vi "Bitfile EST Interfaces.vi"(11 "Version":T1) -> (2 "IP Types":T2[](array[typedef]), 3 "IP Interface":variant[](array[variant]))   [LabVIEW 2019, in "Engine Simulation Toolkit System Explorer.lvlib"]
uses:
  Engine Simulation Toolkit System Explorer.lvlib
  Shared/IP Interface Enum.ctl
  Shared/Bitfile EST Version.ctl
  Shared/Engine Simulation Toolkit Shared.lvlib
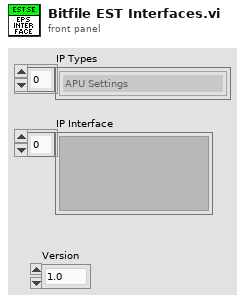
[diagram p1: front panel]
types:
  T1 = typedef "Engine Simulation Toolkit Shared.lvlib/Bitfile EST Version.ctl" = enum16{"1.0", "1.1", "1.2", "1.3", "1.4"}
  T2 = typedef "Engine Simulation Toolkit Shared.lvlib/IP Interface Enum.ctl" = enum16{"APU Settings", "APU Shared Settings", "APU Output", "APU Input", "Analog Replay Settings", "Analog Replay Load Input", "Analog Replay Input", "ETiming Capture Output", "ETiming Meas Settings", "ETiming Meas Output", "Digital PatGen Settings", "Digital PatGen Input", "Digital PatGen Load Input", "Knock Sensor Input", "Knock Sensor Settings", "Knock Cyl Input", "Knock Cyl Settings", "Dir Speed Input", "Dir Speed Settings", "Dir Speed Load Input", "APU Go"}
  T3 = cluster{"acceleration":fxp<+,18,-20>, "max cycle":fxp<+,2,2>, "enable accel":bool}
  T4 = cluster{"acceleration":fxp<+,18,-20>, "enable accel":bool}
  T5 = cluster{"cycle start":fxp<+,2,2>, "crank start":u16, "stuck limit":fxp<+,18,18>}
  T6 = cluster{"start":fxp<+,17,17>, "stuck limit":fxp<+,18,18>}
  T7 = cluster{"crank":u16, "cycle":u16, "actual speed":fxp<+/-,23,2>}
  T8 = cluster{"desired speed":fxp<+/-,23,2>, "reset":bool}
  T9 = cluster{"ReverseNegate":bool, "CycleAngle":bool, "SpeedThreshold":fxp<+/-,23,2>, "AOBelowThreshold":i16}
  T10 = cluster{"Data":i16[], "LoadOffset":u16, "Done":bool}
  T11 = cluster{"Offset":i16, "VScaleSlope":fxp<+,18,6>, "VScaleIntercept":fxp<+/-,18,3>}
  T12 = cluster{"Start":u16, "End":u16, "Duration (tics)":fxp<+,18,18>, "Event present":bool}
  T13 = cluster{"max":u16, "min":u16, "active high":bool, "wrap":bool, "full window":bool}
  T14 = cluster{"max":u16, "min":u16, "active high":bool, "wrap":bool}
  T15 = cluster{"stuck active":bool, "window all active":bool, "window orphan start":bool, "window orphan end":bool}
  T16 = cluster{"edge 1":u16, "edge 2":u16, "cycle angle":bool, "enabled":bool, "first falling":bool}
  T17 = cluster{"edge 1":u16, "edge 2":u16, "cycle angle":bool, "enabled":bool, "first falling":bool, "fault":bool, "fault wrap":bool, "fault value":bool, "fault count":fxp<+,4,4>, "use fault count":bool}
  T18 = cluster{"address":fxp<+,11,11>, "done":bool, "angle":u16}
  T19 = cluster{"low freq (periods/tick)":fxp<+,32,0>, "high freq (periods/tick)":fxp<+,32,0>, "duration (1.25MHz tics)":fxp<+,18,18>, "low freq speed slope":fxp<+,16,-3>, "low freq speed intercept":fxp<+,10,-10>, "low freq by speed":bool}
  T20 = cluster{"probability compare":u16, "high freq scaler":fxp<+,10,0>, "trigger position":u16}
  T21 = cluster{"td (tics)":u16, "tf (tics)":u16, "tr (tics)":u16}
  T22 = cluster{"Upper Value":u16, "Lower Value":u16, "Upper Index":fxp<+,10,10>, "Lower Index":fxp<+,10,10>, "Enabled":bool}
  T23 = cluster{"address":fxp<+,10,10>, "done":bool, "angle":u16}
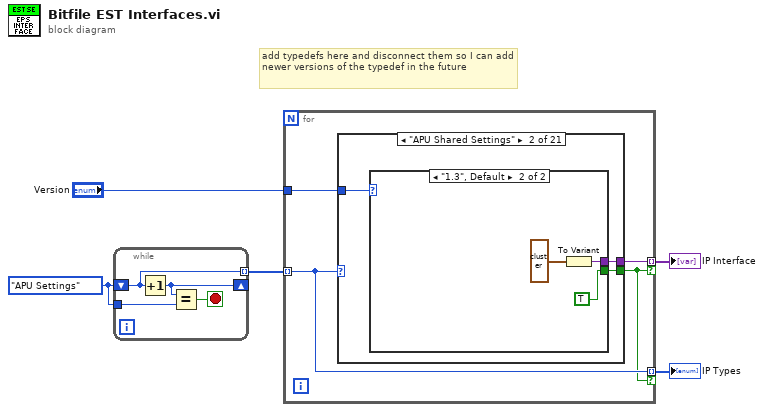
[diagram p0: block diagram]
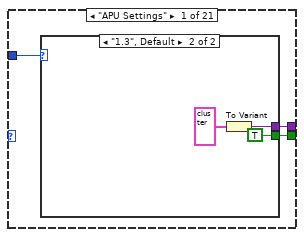
[diagram p2: hidden frame]
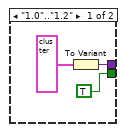
[diagram p3: hidden frame]
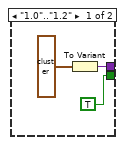
[diagram p4: hidden frame]
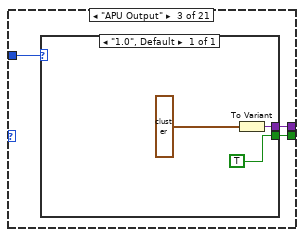
[diagram p5: hidden frame]
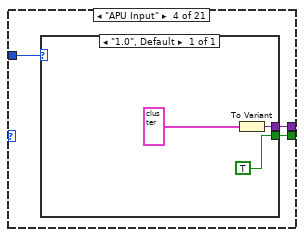
[diagram p6: hidden frame]
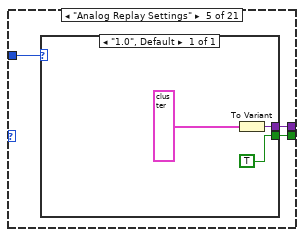
[diagram p7: hidden frame]
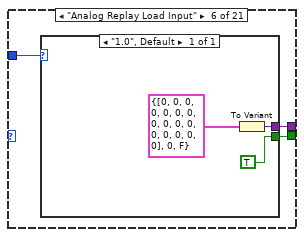
[diagram p8: hidden frame]
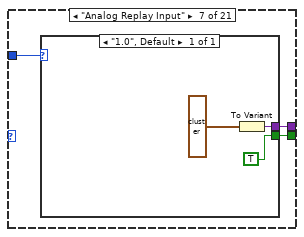
[diagram p9: hidden frame]
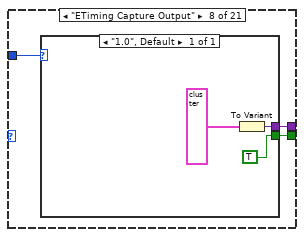
[diagram p10: hidden frame]
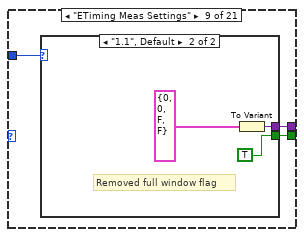
[diagram p11: hidden frame]
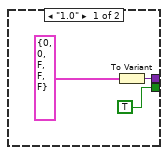
[diagram p12: hidden frame]
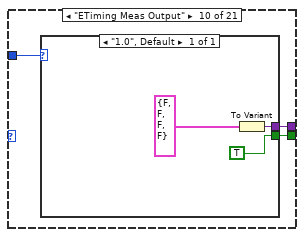
[diagram p13: hidden frame]
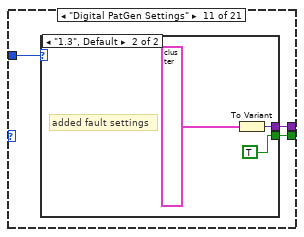
[diagram p14: hidden frame]
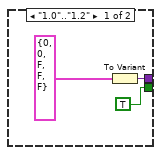
[diagram p15: hidden frame]
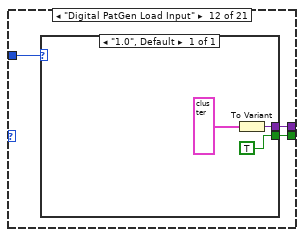
[diagram p16: hidden frame]
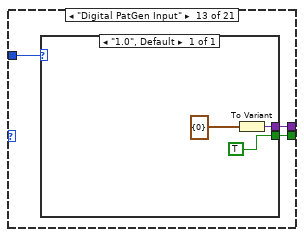
[diagram p17: hidden frame]
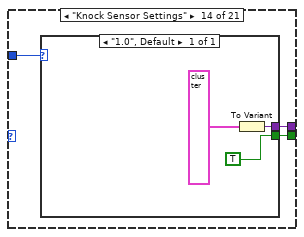
[diagram p18: hidden frame]
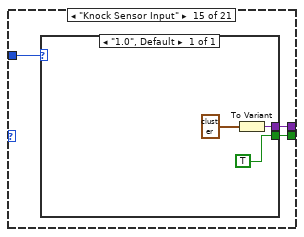
[diagram p19: hidden frame]
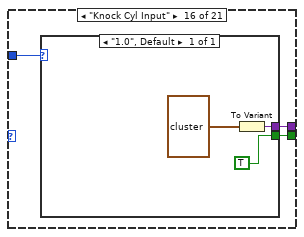
[diagram p20: hidden frame]
diagram:
  w4 = IP_Interface_Enum."APU Settings" ("IP Interface")
  # "add typedefs here and disconnect them so I can add newer versions of the typedef in the future"
  n1 = while {
    shift-right: [w7] -> _
    shift-left: w4 -> [w9]
    tunnel: [w9] -> w3 mode=indexing
    tunnel: w4 -> [w6]
    stop <- w8 stop-if-true
    n2 = Increment(x=w9) -> (x+1=w7:T2)
    n3 = Equal?(x=w7, y=w6) -> (x = y?=w8:bool)
  }
  n4 = for {
    tunnel: w3 -> [w11] mode=indexing
    tunnel: "Version" -> [w13]
    tunnel: [w12] -> w2 mode=indexing if=w10
    tunnel: [w11] -> w1 mode=indexing if=w10
    n5 = case shown="\"APU Shared Settings\"" w11 {
      tunnel: w13 -> [w16 w25 w34 w40 w46 w52 w58 w64 w70 w79 w85 w94 w100 w106 w112 w118 w124 w130 w136 w142 w148]
      tunnel: [w15 w24 w33 w39 w45 w51 w57 w63 w69 w78 w84 w93 w99 w105 w111 w117 w123 w129 w135 w141 w147] -> w12
      tunnel: [w14 w23 w32 w38 w44 w50 w56 w62 w68 w77 w83 w92 w98 w104 w110 w116 w122 w128 w134 w140 w146] -> w10
      frame "APU Settings" {
        n6 = case shown="\"1.3\", Default" w16 {
          tunnel: [w18 w20] -> w15
          tunnel: [TRUE ("done") TRUE ("done")] -> w14
          frame "1.0".."1.2" {
            n7 = To Variant(anything=T3 {"acceleration"=0.0, "max cycle"=0.0, "enable accel"=FALSE}) -> (Variant=w18:variant)
          }
          frame "1.3", Default {
            n8 = To Variant(anything=T4 {"acceleration"=0.0, "enable accel"=FALSE} ("settings with acceleration")) -> (Variant=w20:variant)
          }
        }
      }
      frame "APU Shared Settings" {
        n9 = case shown="\"1.3\", Default" w25 {
          tunnel: [w27 w31] -> w24
          tunnel: [TRUE ("done") TRUE ("done")] -> w23
          frame "1.0".."1.2" {
            n10 = To Variant(anything=T5 {"cycle start"=0.0, "crank start"=0, "stuck limit"=0.0}) -> (Variant=w27:variant)
          }
          frame "1.3", Default {
            n11 = To Variant(anything=T6 {"start"=0.0, "stuck limit"=0.0} ("APU Shared Settings")) -> (Variant=w31:variant)
          }
        }
      }
      frame "APU Output" {
        n12 = case shown="\"1.0\", Default" w34 {
          tunnel: [w37] -> w33
          tunnel: [TRUE ("done")] -> w32
          frame "1.0", Default {
            n13 = To Variant(anything=T7 {"crank"=0, "cycle"=0, "actual speed"=0.0}) -> (Variant=w37:variant)
          }
        }
      }
      frame "APU Input" {
        n14 = case shown="\"1.0\", Default" w40 {
          tunnel: [w43] -> w39
          tunnel: [TRUE ("done")] -> w38
          frame "1.0", Default {
            n15 = To Variant(anything=T8 {"desired speed"=0.0, "reset"=FALSE}) -> (Variant=w43:variant)
          }
        }
      }
      frame "Analog Replay Settings" {
        n16 = case shown="\"1.0\", Default" w46 {
          tunnel: [w49] -> w45
          tunnel: [TRUE ("done")] -> w44
          frame "1.0", Default {
            n17 = To Variant(anything=T9 {"ReverseNegate"=FALSE, "CycleAngle"=FALSE, "SpeedThreshold"=0.0, "AOBelowThreshold"=0}) -> (Variant=w49:variant)
          }
        }
      }
      frame "Analog Replay Load Input" {
        n18 = case shown="\"1.0\", Default" w52 {
          tunnel: [w55] -> w51
          tunnel: [TRUE ("done")] -> w50
          frame "1.0", Default {
            n19 = To Variant(anything=T10 {"Data"=[0, 0, 0, 0, 0, 0, 0, 0, 0, 0, 0, 0, 0, 0, 0, 0], "LoadOffset"=0, "Done"=FALSE}) -> (Variant=w55:variant)
          }
        }
      }
      frame "Analog Replay Input" {
        n20 = case shown="\"1.0\", Default" w58 {
          tunnel: [w61] -> w57
          tunnel: [TRUE ("done")] -> w56
          frame "1.0", Default {
            n21 = To Variant(anything=T11 {"Offset"=0, "VScaleSlope"=0.0, "VScaleIntercept"=0.0}) -> (Variant=w61:variant)
          }
        }
      }
      frame "ETiming Capture Output" {
        n22 = case shown="\"1.0\", Default" w64 {
          tunnel: [w67] -> w63
          tunnel: [TRUE ("done")] -> w62
          frame "1.0", Default {
            n23 = To Variant(anything=T12 {"Start"=0, "End"=0, "Duration (tics)"=0.0, "Event present"=FALSE}) -> (Variant=w67:variant)
          }
        }
      }
      frame "ETiming Meas Settings" {
        n24 = case shown="\"1.1\", Default" w70 {
          tunnel: [w73 w76] -> w69
          tunnel: [TRUE ("done") TRUE ("done")] -> w68
          frame "1.0" {
            n25 = To Variant(anything=T13 {"max"=0, "min"=0, "active high"=FALSE, "wrap"=FALSE, "full window"=FALSE}) -> (Variant=w73:variant)
          }
          frame "1.1", Default {
            # "Removed full window flag"
            n26 = To Variant(anything=T14 {"max"=0, "min"=0, "active high"=FALSE, "wrap"=FALSE}) -> (Variant=w76:variant)
          }
        }
      }
      frame "ETiming Meas Output" {
        n27 = case shown="\"1.0\", Default" w79 {
          tunnel: [w82] -> w78
          tunnel: [TRUE ("done")] -> w77
          frame "1.0", Default {
            n28 = To Variant(anything=T15 {"stuck active"=FALSE, "window all active"=FALSE, "window orphan start"=FALSE, "window orphan end"=FALSE}) -> (Variant=w82:variant)
          }
        }
      }
      frame "Digital PatGen Settings" {
        n29 = case shown="\"1.3\", Default" w85 {
          tunnel: [w88 w91] -> w84
          tunnel: [TRUE ("done") TRUE ("done")] -> w83
          frame "1.0".."1.2" {
            n30 = To Variant(anything=T16 {"edge 1"=0, "edge 2"=0, "cycle angle"=FALSE, "enabled"=FALSE, "first falling"=FALSE} ("settings")) -> (Variant=w88:variant)
          }
          frame "1.3", Default {
            # "added fault settings"
            n31 = To Variant(anything=T17 {"edge 1"=0, "edge 2"=0, "cycle angle"=FALSE, "enabled"=FALSE, "first falling"=FALSE, "fault"=FALSE, "fault wrap"=FALSE, "fault value"=FALSE, "fault count"=0.0, "use fault count"=FALSE} ("settings")) -> (Variant=w91:variant)
          }
        }
      }
      frame "Digital PatGen Load Input" {
        n32 = case shown="\"1.0\", Default" w94 {
          tunnel: [w97] -> w93
          tunnel: [TRUE ("done")] -> w92
          frame "1.0", Default {
            n33 = To Variant(anything=T18 {"address"=0.0, "done"=FALSE, "angle"=0}) -> (Variant=w97:variant)
          }
        }
      }
      frame "Digital PatGen Input" {
        n34 = case shown="\"1.0\", Default" w100 {
          tunnel: [w103] -> w99
          tunnel: [TRUE ("done")] -> w98
          frame "1.0", Default {
            n35 = To Variant(anything=cluster{"Offset":i16} {"Offset"=0}) -> (Variant=w103:variant)
          }
        }
      }
      frame "Knock Sensor Settings" {
        n36 = case shown="\"1.0\", Default" w106 {
          tunnel: [w109] -> w105
          tunnel: [TRUE ("done")] -> w104
          frame "1.0", Default {
            n37 = To Variant(anything=T19 {"low freq (periods/tick)"=0.0, "high freq (periods/tick)"=0.0, "duration (1.25MHz tics)"=0.0, "low freq speed slope"=0.0, "low freq speed intercept"=0.0, "low freq by speed"=FALSE}) -> (Variant=w109:variant)
          }
        }
      }
      frame "Knock Sensor Input" {
        n38 = case shown="\"1.0\", Default" w112 {
          tunnel: [w115] -> w111
          tunnel: [TRUE ("done")] -> w110
          frame "1.0", Default {
            n39 = To Variant(anything=cluster{"low freq scaler":fxp<+,10,0>} {"low freq scaler"=0.0} ("settings")) -> (Variant=w115:variant)
          }
        }
      }
      frame "Knock Cyl Input" {
        n40 = case shown="\"1.0\", Default" w118 {
          tunnel: [w121] -> w117
          tunnel: [TRUE ("done")] -> w116
          frame "1.0", Default {
            n41 = To Variant(anything=T20 {"probability compare"=65535, "high freq scaler"=0.0, "trigger position"=0} ("input")) -> (Variant=w121:variant)
          }
        }
      }
      frame "Knock Cyl Settings" {
        n42 = case shown="\"1.0\", Default" w124 {
          tunnel: [w127] -> w123
          tunnel: [TRUE ("done")] -> w122
          frame "1.0", Default {
            n43 = To Variant(anything=cluster{"seed":u16, "reset":bool} {"seed"=0, "reset"=FALSE} ("settings")) -> (Variant=w127:variant)
          }
        }
      }
      frame "Dir Speed Input" {
        n44 = case shown="\"1.0\", Default" w130 {
          tunnel: [w133] -> w129
          tunnel: [TRUE ("done")] -> w128
          frame "1.0", Default {
            n45 = To Variant(anything=T21 {"td (tics)"=0, "tf (tics)"=0, "tr (tics)"=0} ("settings")) -> (Variant=w133:variant)
          }
        }
      }
      frame "Dir Speed Settings" {
        n46 = case shown="\"1.0\", Default" w136 {
          tunnel: [w139] -> w135
          tunnel: [TRUE ("done")] -> w134
          frame "1.0", Default {
            n47 = To Variant(anything=T22 {"Upper Value"=0, "Lower Value"=0, "Upper Index"=0.0, "Lower Index"=0.0, "Enabled"=FALSE} ("settings")) -> (Variant=w139:variant)
          }
        }
      }
      frame "Dir Speed Load Input" {
        n48 = case shown="\"1.0\", Default" w142 {
          tunnel: [w145] -> w141
          tunnel: [TRUE ("done")] -> w140
          frame "1.0", Default {
            n49 = To Variant(anything=T23 {"address"=0.0, "done"=FALSE, "angle"=0} ("settings")) -> (Variant=w145:variant)
          }
        }
      }
      frame "APU Go" {
        n50 = case shown="\"1.1\", Default" w148 {
          tunnel: [w151 _] -> w147
          tunnel: [TRUE ("done") _] -> w146
          frame "1.1", Default {
            n51 = To Variant(anything=FALSE ("done")) -> (Variant=w151:variant)
          }
          frame "1.0" {
            # "Did not exist in 1.0"
          }
        }
      }
    }
  }
  "IP Types" <- w1
  "IP Interface" <- w2
